vi "Get App Kind, Name & Path.vi"(8 "Error In":errorcluster, 11 "Callling VI Path":path) -> (0 "Error Out":errorcluster, 1 "Application Path":path, 2 "Application:Name":string, 3 "Application:Kind":T1(ring))   [LabVIEW 2021, in "Utilities.lvlib"]
uses:
  Utilities.lvlib
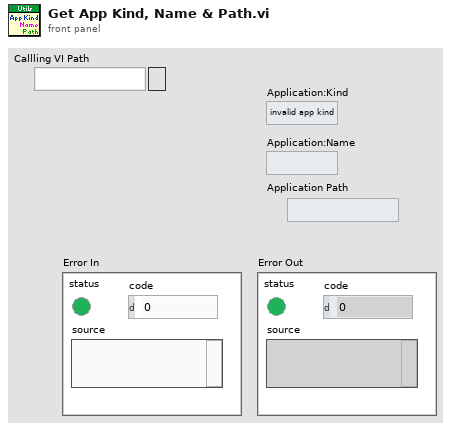
[diagram p1: front panel]
types:
  T1 = enum32{"invalid app kind", "Development System", "Run Time System", "Student Edition", "Embedded LabVIEW", "Evaluation", "Custom"}
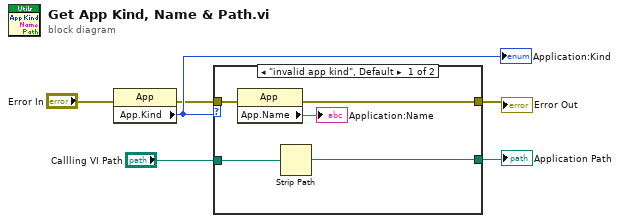
[diagram p0: block diagram]
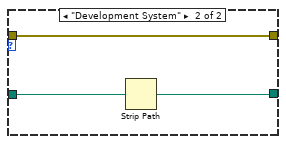
[diagram p2: hidden frame]
diagram:
  n1 = property class="App"(error in="Error In") -> (error out=w3:errorcluster, "App.Kind"=w6:T1)  [unwired: 1 in, 1 out]
  "Application:Kind" <- w6
  n2 = case shown="\"invalid app kind\", Default" w6 {
    tunnel: "Callling VI Path" -> [w8 w14]
    tunnel: [w7 w12] -> w5
    tunnel: w3 -> [w11 w13]
    tunnel: [w10 w13] -> w2
    frame "invalid app kind", Default {
      n3 = property class="App"(error in=w11) -> (error out=w10:errorcluster, "App.Name"=→"Application:Name":string)  [unwired: 1 in, 1 out]
      n4 = Strip Path(path=w8) -> (stripped path=w7:path)  [unwired: 1 out]
    }
    frame "Development System" {
      n5 = Strip Path(path=w14) -> (stripped path=w12:path)  [unwired: 1 out]
    }
  }
  "Application Path" <- w5
  "Error Out" <- w2
